vi "S2C_CMD_ParseCmd.vi"(8 "Error In":errorcluster, 11 "Settings":T1) -> (0 "Error Out":errorcluster, 1 "Returns":string[](array[string]), 2 "Parameters":string[][](array[string]), 3 "Commands":string[](array[string]), 4 "RtnIndex":i32, 5 "CmdIndex":i32)   [LabVIEW 2015]
doc: "Formats the input settings and looks up the Commands, Returns, and Parameters."
uses:
  S2C_CMD_Globals.vi
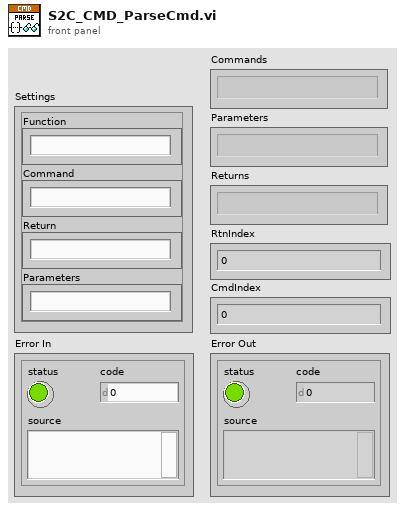
[diagram p1: front panel]
types:
  T1 = cluster{"Function":string, "Command":string, "Return":string, "Parameters":string}
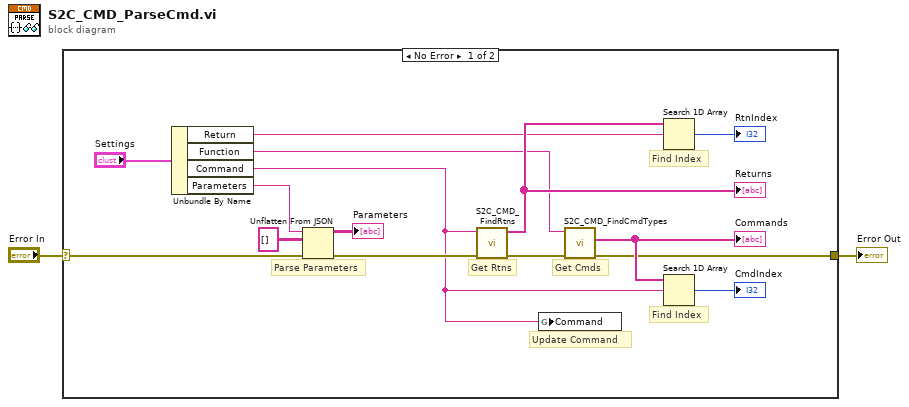
[diagram p0: block diagram]
diagram:
  n1 = case shown="No Error" "Error In" {
    selector: "Error In" -> [w13 w18]
    tunnel: [w11 w18] -> w1
    frame No Error {
      # "Get Rtns"
      # "Find Index"
      # "Parse Parameters"
      # "Find Index"
      # "Update Command"
      # "Get Cmds"
      n2 = Unbundle By Name("Settings") -> ("Return"=w4:string, "Function"=w3:string, "Command"=w5:string, "Parameters"=w6:string)
      n3 = Unflatten From JSON(JSON string=w6, type and defaults=string[][] [], error in (no error)=w13) -> (value=→"Parameters":string[][], error out=w10:errorcluster)  [unwired: 4 in]
      n4 = call "S2C_CMD_FindRtns.vi"("Error In"=w10, "Command"=w5) -> ("Error Out"=w9:errorcluster, "AllRtns"=w8:string[])  [unwired: 8 in]
      "Returns" <- w8
      n5 = global write "S2C_CMD_Globals.vi" "Command"(w5) -> ()
      n6 = call "S2C_CMD_FindCmdTypes.vi"("Error In"=w9, "Command"=w3) -> ("Error Out"=w11:errorcluster, "AllCmds"=w17:string[])  [unwired: 7 in, 1 out]
      "Commands" <- w17
      n7 = Search 1D Array(1D array=w8, element=w4) -> (index of element=→"RtnIndex":i32)  [unwired: 1 in]
      n8 = Search 1D Array(1D array=w17, element=w5) -> (index of element=→"CmdIndex":i32)  [unwired: 1 in]
    }
    frame Error {
    }
  }
  "Error Out" <- w1
